vi "XML429_Database_CloseRefnum.vi"(0 "XMLRefnum":refnum<k20>, 11 "Error in":errorcluster) -> (15 "Error out":errorcluster)   [LabVIEW 2015, in "AIT 429 System Explorer.lvlib"]
doc: "XML429_Database_CloseRefnum"
uses:
  <vilib>/xml/Close Reference(Node).vi
  AIT 429 System Explorer.lvlib
  <vilib>/xml/NI_XML.lvlib
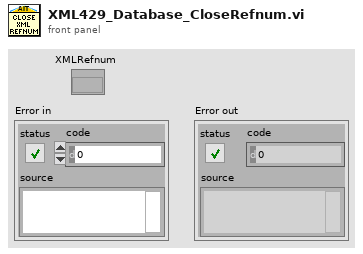
[diagram p1: front panel]
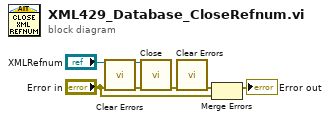
[diagram p0: block diagram]
diagram:
  n1 = call <vilib>:"Clear Errors.vi"("error in (no error)"="Error in") -> ("error out"=w6:errorcluster)  [unwired: 5 in, 1 out]
  n2 = call-poly <vilib>:"Close.vi"("error in (no error)"=w6, "node"="XMLRefnum") -> ("error out"=w4:errorcluster)  [unwired: 7 in]
  n3 = call <vilib>:"Clear Errors.vi"("error in (no error)"=w4) -> ("error out"=w2:errorcluster)  [unwired: 5 in, 1 out]
  n4 = Merge Errors(w2, "Error in") -> (→"Error out":errorcluster)
